vi "Header or Footer vertical margin.vi"(0 "PDF Report IN":refnum<class "PDF Report Class.lvclass">, 2 "Vertical margin":dbl=-1.0, 11 "error in (no error)":errorcluster, 13 "Position":T1=enum."Footer") -> (4 "PDF Report OUT":refnum<class "PDF Report Class.lvclass">, 15 "error out":errorcluster)   [LabVIEW 2019]
doc: "Version 1.1\nDeveloped by Jean-Marc Simard\nCopyright © 2012, Exaprom Inc.\nAll rights reserved.\nLicense: BSD\n\nWith iTextSharp 4.1.6 (http://itextsharp.sourceforge.net)\nunder Mozilla Public License Version 1.1\n(http://www.mozilla.org/MPL/MPL-1.1.html)"
uses:
  <userlib>/Exaprom PDF/LV Class/PDF Report Class/PDF Report Class.lvclass
  <userlib>/Exaprom PDF/Controls/Header, Footer and Watermark Controls/Header or Footer.ctl
  C:/Program Files/National Instruments/LabVIEW 2019/user.lib/Exaprom PDF/DLL/itextsharp.dll
  DLL/itextsharp.dll
  <userlib>/Exaprom PDF/LV Class/Header and Footer Class/Header and Footer Class.lvclass
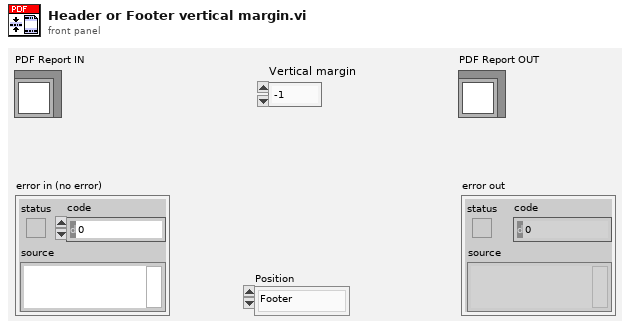
[diagram p1: front panel]
types:
  T1 = typedef "Header or Footer.ctl" = enum16{"Header", "Footer"}
  T2 = typedef "Unit.ctl" = enum16{"inch", "mm"}
  T3 = typedef "Header Footer [ ] V2.ctl" = T4[]
  T4 = typedef "Header Footer cluster V2.ctl" = cluster{"Header or Footer":T1, "Start page":i32, "Start with #":i32, "Type":T5, "Alignment":T6, "Vertical Alignement":T7, "Line spacing":T8, "Image (%)":sgl, "Page #":T9, "Text":string, "Path":string, "Font":T10, "Font refnum":refnum<k24>, "Line":cluster{"Line":T15, "Thickness (points)":sgl, "Colour":T12}, "Vert margin":dbl, "Hyperlink":string}
  T5 = typedef "Header Footer Type.ctl" = enum16{"Select", "Text", "Text + hyperlink", "Page number", "Image", "Image + hyperlink"}
  T6 = typedef "Header footer horiz alignment.ctl" = enum16{"Left", "Center", "Right"}
  T7 = typedef "Cell Vertical alignment.ctl" = enum16{"TOP", "MIDDLE", "BOTTOM"}
  T8 = typedef "Line spacing.ctl" = enum16{"Select", "1.0", "1.5", "2.0"}
  T9 = typedef "Page number.ctl" = cluster{"Text 1":string, "Text 2":string, "Text 3":string}
  T10 = typedef "Font complete cluster horizontal.ctl" = cluster{"Name":string, "Size":T11, "Color":T12, "Style":cluster{"Bold":bool, "Italic":bool, "Underline":bool, "Strikeout":bool}, "Type":T13}
  T11 = typedef "Font size.ctl" = sgl
  T12 = typedef "Font color.ctl" = u32
  T13 = typedef "Type and encoding.ctl" = cluster{"Type&direction":T14, "Embedded":bool, "Encoding":string}
  T14 = typedef "Type and run direction.ctl" = enum16{"Select", "ASCII", "UTF-16", "UTF-16 (default)", "UTF-16 (LTR)", "UTF-16 (RTL)"}
  T15 = typedef "Header Footer Line.ctl" = enum16{"No line", "Horizontal line"}
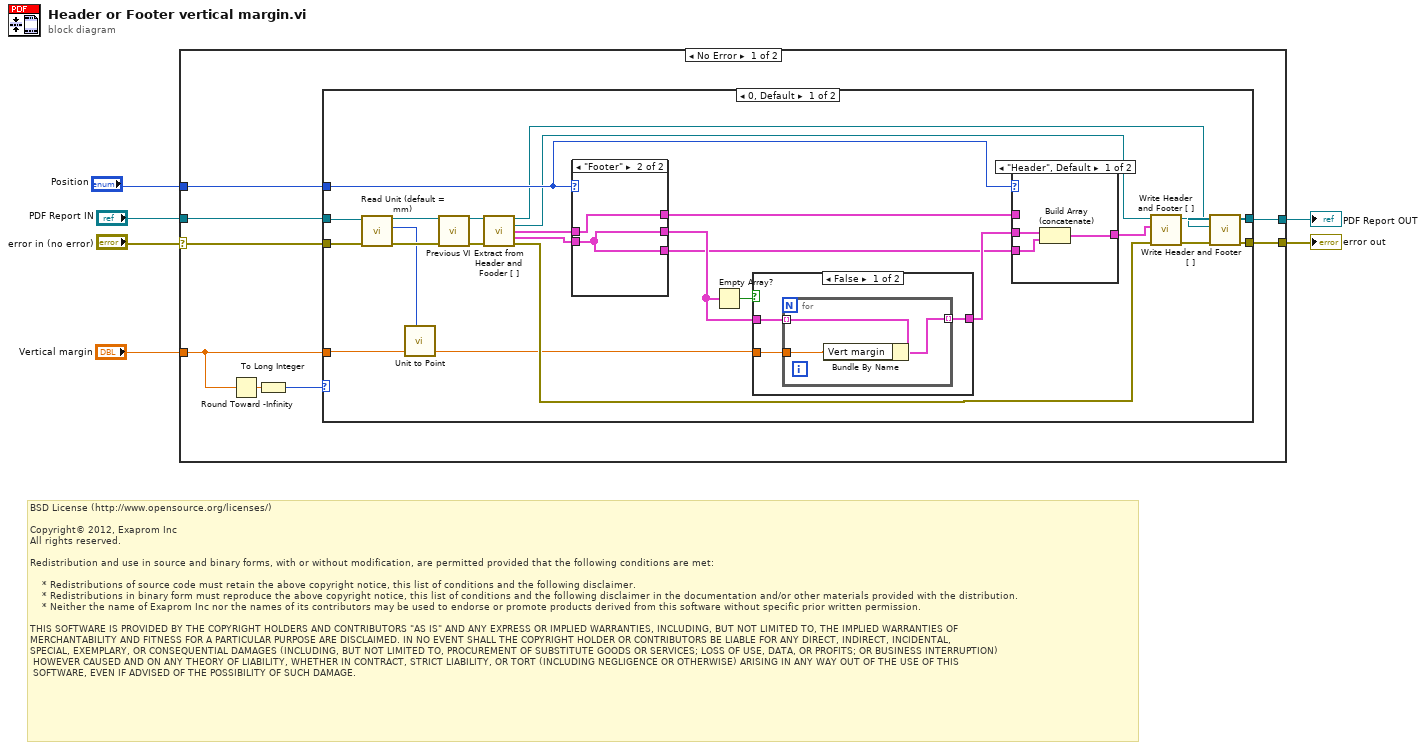
[diagram p0: block diagram]
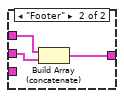
[diagram p4: hidden frame]
diagram:
  # "BSD License (http://www.opensource.org/licenses/)\n\nCopyright© 2012, Exaprom Inc\nAll rights reserved.\n\nRedistribution and use in source and binary forms, with or without modification, are permitted provided that the following conditions are met:\n\n    * Redistributions of source code must retain the above copyright notice, this list of conditions and the following disclaimer.\n    * Redistributions in binary form must reproduce the above copyright notice, this list of conditions and the following disclaimer in the documentation and/or other materials provided with the distribution.\n    * Neither the name of Exaprom Inc nor the names of its contributors may be used to endorse or promote products derived from this software without specific prior written permission.\n\nTHIS SOFTWARE IS PROVIDED BY THE COPYRIGHT HOLDERS AND CONTRIBUTORS \"AS IS\" AND ANY EXPRESS OR IMPLIED WARRANTIES, INCLUDING, BUT NOT LIMITED TO, THE IMPLIED WARRANTIES OF \nMERCHANTABILITY AND FITNESS FOR A PARTICULAR PURPOSE ARE DISCLAIMED. IN NO EVENT SHALL THE COPYRIGHT HOLDER OR CONTRIBUTORS BE LIABLE FOR ANY DIRECT, INDIRECT, INCIDENTAL,\nSPECIAL, EXEMPLARY, OR CONSEQUENTIAL DAMAGES (INCLUDING, BUT NOT LIMITED TO, PROCUREMENT OF SUBSTITUTE GOODS OR SERVICES; LOSS OF USE, DATA, OR PROFITS; OR BUSINESS INTERRUPTION)\n HOWEVER CAUSED AND ON ANY THEORY OF LIABILITY, WHETHER IN CONTRACT, STRICT LIABILITY, OR TORT (INCLUDING NEGLIGENCE OR OTHERWISE) ARISING IN ANY WAY OUT OF THE USE OF THIS\n SOFTWARE, EVEN IF ADVISED OF THE POSSIBILITY OF SUCH DAMAGE."
  n1 = case shown="No Error" "error in (no error)" {
    selector: "error in (no error)" -> [w13 w58]
    tunnel: "PDF Report IN" -> [w14 w59]
    tunnel: "Position" -> [w12 _]
    tunnel: [w10 w59] -> w2
    tunnel: "Vertical margin" -> [w7 _]
    tunnel: [w11 w58] -> w3
    frame No Error {
      n2 = Round Toward -Infinity(1:w7) -> (0:w9:dbl)
      n3 = To Long Integer(number=w9) -> (32bit integer=w8:i32)
      n4 = case shown="0, Default" w8 {
        tunnel: w14 -> [w20 w57]
        tunnel: w13 -> [w19 w56]
        tunnel: w7 -> [w16 _]
        tunnel: w12 -> [w35 _]
        tunnel: [w24 w56] -> w11
        tunnel: [w23 w57] -> w10
        frame 0, Default {
          n5 = call-dynamic "Read Unit (default = mm).vi"("error in (no error)"=w19, "PDF Report Class in"=w20) -> ("error out"=w18:errorcluster, "Unit (default = mm)"=w17:T2, "PDF Report Class out"=w21:refnum<class "PDF Report Class.lvclass">)  [unwired: 7 in]
          n6 = call <userlib>:"Unit to Point.vi"("X unit"=w16, "Unit (default = mm)"=w17) -> ("X point"=w15:sgl)  [unwired: 7 out]
          n7 = call <userlib>:"Previous VI.vi"("PDF Report IN"=w21, "error in (no error)"=w18) -> ("PDF Report OUT"=w37:refnum<class "PDF Report Class.lvclass">, "error out"=w36:errorcluster)  [unwired: 12 out]
          n8 = call <userlib>:"Extract from Header and Fooder [ ].vi"("PDF Report IN"=w37, "error in (no error)"=w36) -> ("PDF Report OUT"=w22:refnum<class "PDF Report Class.lvclass">, "Header and Footer duplicate"=w29:refnum<class "Header and Footer Class.lvclass">, "Header [ ]"=w34:T3, "Footer [ ]"=w33:T3, "error out"=w27:errorcluster)  [unwired: 9 in]
          n9 = case shown="\"Footer\"" w35 {
            tunnel: w34 -> [w40 w42]
            tunnel: [w40 w41] -> w32
            tunnel: w33 -> [_ w41]
            tunnel: [_ w42] -> w31
            tunnel: [_ w41] -> w30
            frame "Header", Default {
            }
            frame "Footer" {
            }
          }
          n10 = Empty Array?(array=w32) -> (empty?=w38:bool)
          n11 = case shown="False" w38 {
            tunnel: w15 -> [w45 _]
            tunnel: w32 -> [w44 w49]
            tunnel: [w43 w49] -> w39
            frame False {
              n12 = for {
                tunnel: w45 -> [w48]
                tunnel: w44 -> [w47] mode=indexing
                tunnel: [w46] -> w43 mode=indexing
                n13 = Bundle By Name(cluster=w47, "Vert margin"=w48) -> (w46:T4)
              }
            }
            frame True {
            }
          }
          n14 = case shown="\"Header\", Default" w35 {
            tunnel: w39 -> [w52 w54]
            tunnel: w31 -> [_ w55]
            tunnel: w30 -> [w51 _]
            tunnel: [w50 w53] -> w28
            frame "Header", Default {
              n15 = Build Array (concatenate)(w52, w51) -> (w50:T3)
            }
            frame "Footer" {
              n16 = Build Array (concatenate)(w55, w54) -> (w53:T3)
            }
          }
          n17 = call-dynamic "Write Header and Footer [ ].vi"("error in (no error)"=w27, "Header and Footer [ ]"=w28, "Header and Footer Class in"=w29) -> ("error out"=w25:errorcluster, "Header and Footer Class out"=w26:refnum<class "Header and Footer Class.lvclass">)  [unwired: 7 in]
          n18 = call-dynamic "Write Header and Footer [ ].vi"("error in (no error)"=w25, "Header and Footer Class.lvclass"=w26, "PDF Report Class in"=w22) -> ("error out"=w24:errorcluster, "PDF Report Class out"=w23:refnum<class "PDF Report Class.lvclass">)  [unwired: 7 in]
        }
        frame ..-1 {
        }
      }
    }
    frame Error {
    }
  }
  "PDF Report OUT" <- w2
  "error out" <- w3
